vi "color.vi"(8 "Error In":errorcluster, 11 "QBrush In":refnum<class "QBrush.lvclass">) -> (0 "Error Out":errorcluster, 2 "Value":refnum<class "QColor.lvclass">, 3 "QBrush Out":refnum<class "QBrush.lvclass">)   [LabVIEW 2014, in "QBrush.lvclass"]
doc: "LabVIEW-specific documentation is not yet available. See <b>http://doc.qt.io/qt-5/QBrush.html#color</b>"
uses:
  QBrush.lvclass
  QColor/QColor.lvclass
  LQ Core/LQSerialData/LQSerialData.lvclass/LQSerialData.ctl
  LQ Core/LQ Core.lvlib
  LQ Core/LQSerialData/LQSerialData.lvclass
panel:
  # "Copyright (c) 2016 Sze Howe Koh\n\nThis Source Code Form is subject to the terms of the Mozilla Public\nLicense, v. 2.0. If a copy of the MPL was not distributed with this\nfile, You can obtain one at http://mozilla.org/MPL/2.0/."
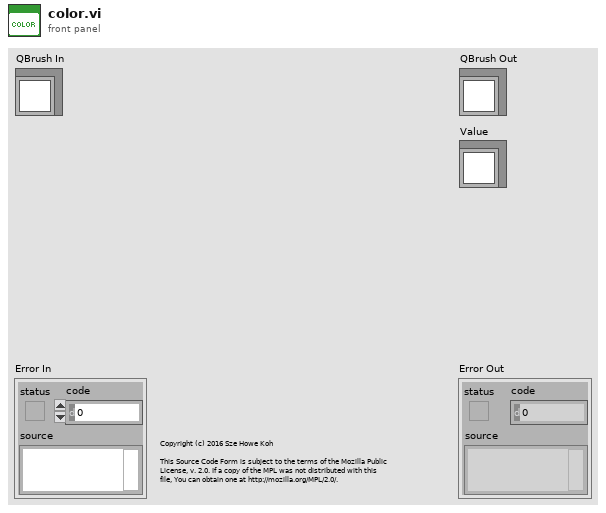
[diagram p1: front panel]
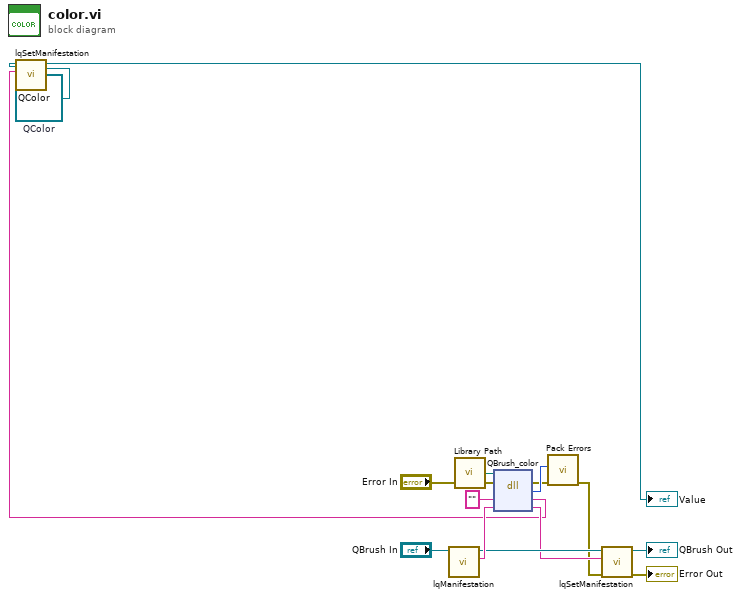
[diagram p0: block diagram]
diagram:
  w1 = refnum<class "QColor.lvclass"> refnum  # QColor
  n1 = call "lqManifestation.vi"("LQSerialData in"="QBrush In") -> ("Manifestation"=w13:string, "LQSerialData out"=w11:refnum<class "QBrush.lvclass">)  [unwired: 9 in]
  n2 = call "Library Path.vi"() -> ("Library Path"=w8:path)
  n3 = dll-call lib="?" fn="QBrush_color"(path in=w8, error in="Error In", "_retVal"="" ("retVal"), "_instance"=w13) -> (error out=w5:errorcluster, w6:i32, "_retVal"=w2:string, "_instance"=w9:string)  [unwired: 1 in, 1 out]
  n4 = call "lqSetManifestation.vi"("Manifestation"=w2, "LQSerialData in"=w1) -> ("LQSerialData out"=→"Value":refnum<class "QColor.lvclass">)  [unwired: 8 in, 1 out]
  n5 = call "Pack Errors.vi"("Error In"=w5, "Error Code"=w6) -> ("Error Out"=w4:errorcluster)  [unwired: 9 in]
  n6 = call "lqSetManifestation.vi"("Error In"=w4, "Manifestation"=w9, "LQSerialData in"=w11) -> ("Error Out"=→"Error Out":errorcluster, "LQSerialData out"=→"QBrush Out":refnum<class "QBrush.lvclass">)  [unwired: 7 in]
